vi "helpSamplingInterval.vi"   [LabVIEW 2020, in "main.lvlib"]
uses:
  main.lvlib
panel:
  # "Changing the sampling interval clears the graph.\nAcquired data is always averaged over 1 s.\nIf the sampling interval is set to a value greater than 1 s,\nthe graph is updated at intervals equal to the selected sampling interval;\nhowever, each displayed point and each value saved to file is still\naveraged over 1 s, regardless of the selected sampling interval."
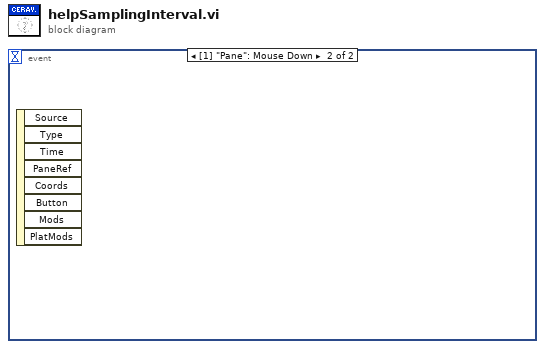
[diagram p0: block diagram]
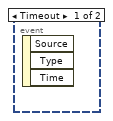
[diagram p2: hidden frame]
diagram:
  n1 = event shown="[1] \"Pane\": Mouse Down" {
    selector: _ -> [_ _]
    dyn-events: _ -> [_ _]
    timeout: _ -> [_ _]
    event Timeout {
      n2 = event-data() -> ()  [unwired: 1 in, 3 out]
    }
    event Mouse Down {
      n3 = event-data() -> ()  [unwired: 1 in, 8 out]
    }
  }
